vi "IBM4_Open.vi"(9 "Mode":enum16{"DC", "AC"}(ring), 11 "COM Port":refnum<visa-resource-name>) -> (0 "error out":errorcluster, 2 "UCC Revision #":string, 3 "COM resource out":refnum<visa-resource-name>)   [LabVIEW 2022 SP3, in "IBM4.lvlib"]
doc: "This VI is used to open the IBM4 (Itsybitsy M4). This should always be the first VI called, when communicating with the IBM4. \n\nThe COM Port must be the correct one for the IBM4, or else an error will be returned. In addition, if the IBM4 has not been loaded with the correct Circuit Python code, an error will also be generated.\n\nIf a properly configure IBM4 exists at that port, then the UCC Revision # will be returned.\n\nRemember to also close the device at the end. If this is not done, you may need to reboot your computer to free up resources."
uses:
  <instrlib>/IBM4/IBM4.lvlib
  <vilib>/Instr/_visa.llb/VISA Configure Serial Port (Instr).vi
panel:
  out "The Mode returned":string
  out "read buffer":string
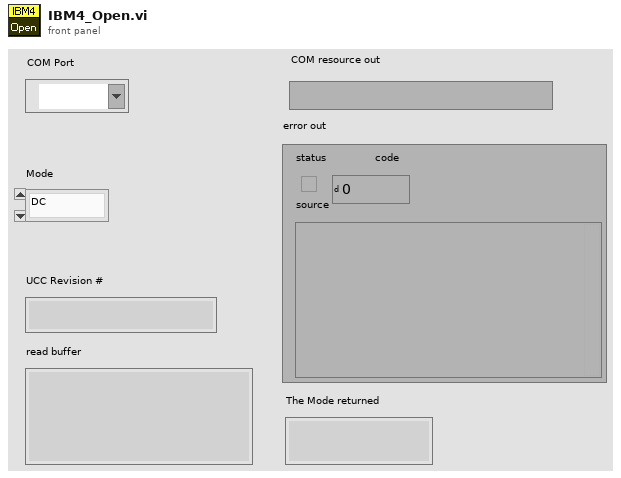
[diagram p1: front panel]
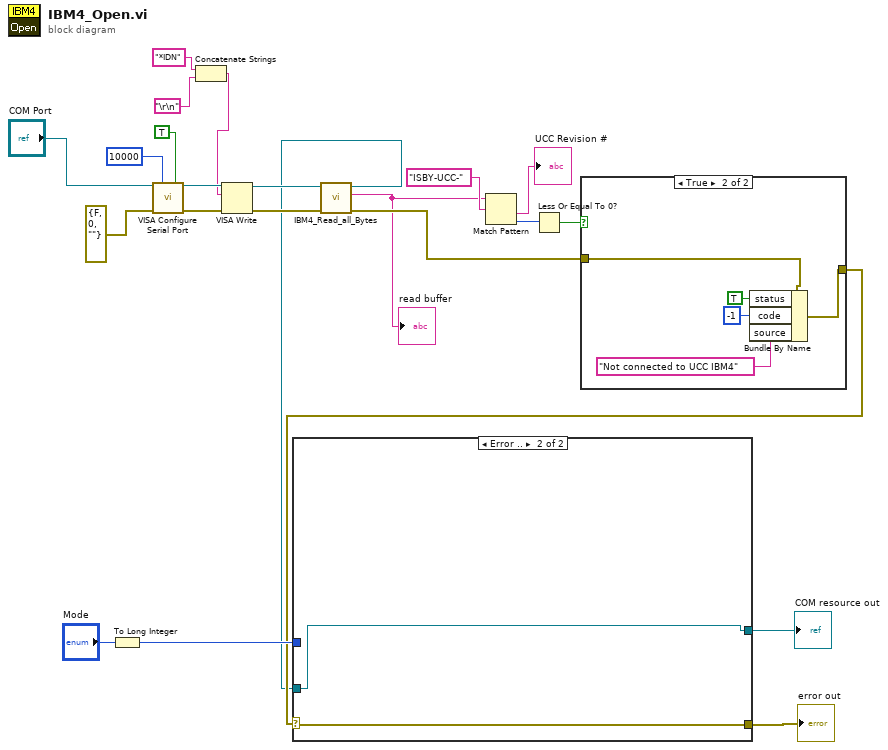
[diagram p0: block diagram]
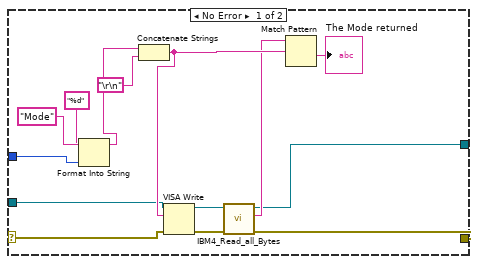
[diagram p2: hidden frame]
diagram:
  n1 = To Long Integer(number="Mode") -> (32bit integer=w8:i32)
  n2 = call-poly "VISA Configure Serial Port"("VISA resource name"="COM Port", "timeout (10sec)"=u32 10000, "Enable Termination\nChar (T)"=TRUE ("Enable Termination\nChar (T)"), "error in (no error)"=errorcluster {"status"=FALSE, "code"=0, "source"=""}) -> ("VISA resource name out"=w20:refnum<visa-resource-name>, "error out"=w19:errorcluster)  [unwired: 10 in]
  n3 = Concatenate Strings("*IDN" ("write buffer"), "\r\n") -> (w16:string)
  n4 = VISA Write(VISA resource name=w20, write buffer=w16, error in (no error)=w19) -> (VISA resource name out=w7:refnum<visa-resource-name>, error out=w6:errorcluster)  [unwired: 1 out]
  n5 = call <instrlib>:"IBM4_Read_all_Bytes.vi"("error in (no error)"=w6, "VISA Refnum in"=w7) -> ("error out"=w4:errorcluster, "String"=w2:string, "VISA Refnum out"=w3:refnum<visa-resource-name>)  [unwired: 3 in]
  "read buffer" <- w2
  n6 = Match Pattern(string=w2, regular expression="ISBY-UCC-" ("format string")) -> (after substring=→"UCC Revision #":string, offset past match=w13:i32)  [unwired: 1 in, 2 out]
  n7 = Less Or Equal To 0?(x=w13) -> (x <= 0?=w12:bool)
  n8 = case shown="True" w12 {
    tunnel: [w24 w28] -> w5
    tunnel: w4 -> [w24 w25]
    frame False {
    }
    frame True {
      n9 = Bundle By Name(cluster=w25, "status"=TRUE, "code"=-1, "source"="Not connected to UCC IBM4") -> (w28:errorcluster)
    }
  }
  n10 = case shown="Error .." w5 {
    selector: w5 -> [w42 w45]
    tunnel: [w32 w45] -> w10
    tunnel: w8 -> [w39 _]
    tunnel: w3 -> [w35 w44]
    tunnel: [w30 w44] -> w1
    frame No Error {
      n11 = Format Into String(format string="%d", initial string="Mode" ("write buffer"), w39) -> (resulting string=w38:string)  [unwired: 1 in, 1 out]
      n12 = Concatenate Strings(w38, "\r\n") -> (w37:string)
      n13 = VISA Write(VISA resource name=w35, write buffer=w37, error in (no error)=w42) -> (VISA resource name out=w34:refnum<visa-resource-name>, error out=w33:errorcluster)  [unwired: 1 out]
      n14 = call <instrlib>:"IBM4_Read_all_Bytes.vi"("error in (no error)"=w33, "VISA Refnum in"=w34) -> ("error out"=w32:errorcluster, "String"=w31:string, "VISA Refnum out"=w30:refnum<visa-resource-name>)  [unwired: 3 in]
      n15 = Match Pattern(string=w31, regular expression=w37) -> (after substring=→"The Mode returned":string)  [unwired: 1 in, 3 out]
    }
    frame Error {
    }
  }
  "error out" <- w10
  "COM resource out" <- w1
